vi "Write_NetworkStream_OCU_Override.vi"(0 "VKey":T1, 5 "Mainsail Position":T4, 7 "Jib Position":T3, 9 "Rudder Setpoint":T2 min=-0.95 max=0.95 scale=1.0..-1.0, 11 "error in (no error)":errorcluster, 12 "OverrideMode":T5) -> (4 "Main Position":T4, 6 "Jib Position":T3, 8 "Rudder Position":T2 min=-0.95 max=0.95 scale=1.0..-1.0, 10 "data string":string, 15 "error out":errorcluster)   [LabVIEW 2013]
doc: "Takes in the key value pressed and changes the value of the main sail, jib, and rudder accordingly with the following mapping of the arrow keys (ish):\n\n\"Page Up\" -- rudder right | \"Up\" -- Main out | \"Page Down\" -- Jib out\n\"Left\" -- rudder left | \"Down\" -- Main in | \"Right\" -- Jib in\n\nIt then bundles the main sail, jib sail, and rudder override commands and sends them to the boat using NetworkStreams. It also bundles with them the override mode so the Forebrain Sense can determine which actuator setting so implement and which to ignore. Deals with coersions, becaues humans can be silly.\n\n\n\nWritten by Victoria Coleman 04/12/14"
uses:
  cRIO_Code/Data/TypeDefs/Sail Set Suggestions.ctl
  cRIO_Code/Data/TypeDefs/OverrideMode.ctl
  cRIO_Code/Data/TypeDefs/MainsailPositionIndicator.ctl
  cRIO_Code/Data/TypeDefs/JibPositionIndicator.ctl
  cRIO_Code/Data/TypeDefs/Rudder Set Suggestions.ctl
  <vilib>/event_ctls.llb/eventvkey.ctl
  cRIO_Code/Data/TypeDefs/OverrideInformation.ctl
  OCU/CommandMessages.ctl
panel:
  in  "Sail Suggesstions":T6 {"MainSailSuggestion" min=0.0 max=1.0; "JibSailSuggestion" min=0.0 max=1.0}
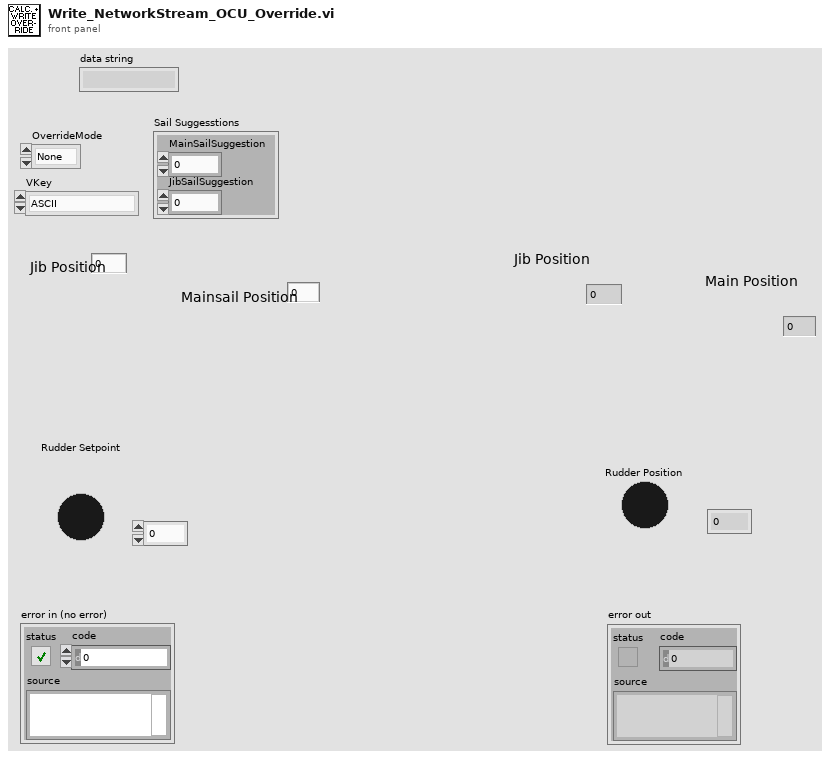
[diagram p1: front panel]
types:
  T1 = typedef "eventvkey.ctl" = enum16{"ASCII", "Enter", "Return", "Shift", "Ctrl", "Alt", "Cmd", "Opt", "Caps", "NumLock", "Clear", "Break", "Up", "Down", "Left", "Right", "Insert", "Delete", "Home", "End", "PageUp", "PageDown", "Escape", "Help", "Pause", "ScrollLock", "F1", "F2", "F3", "F4", "F5", "F6", "F7", "F8", "F9", "F10", "F11", "F12", "F13", "F14", "F15", "F16", "F17", "F18", "F19", "F20", "F21", "F22", "F23", "F24", "Play", "VolumeUp", "VolumeDown", "Mute", "Two Byte Char"}
  T2 = typedef "Rudder Set Suggestions.ctl" = dbl
  T3 = typedef "JibPositionIndicator.ctl" = dbl
  T4 = typedef "MainsailPositionIndicator.ctl" = dbl
  T5 = typedef "OverrideMode.ctl" = enum16{"None", "Rudder", "Sails", "Both"}
  T6 = typedef "Sail Set Suggestions.ctl" = cluster{"MainSailSuggestion":dbl, "JibSailSuggestion":dbl}
  T7 = typedef "OverrideInformation.ctl" = cluster{"OverrideMode":T5, "SailSetting":T6, "Rudder Setpoint":T2, "Sim_Wind_Speed":dbl, "Sim_Wind_Heading":dbl}
  T8 = typedef "CommandMessages.ctl" = enum16{"Pass", "OverrideMode", "Add mission", "Delete mission", "Change constants"}
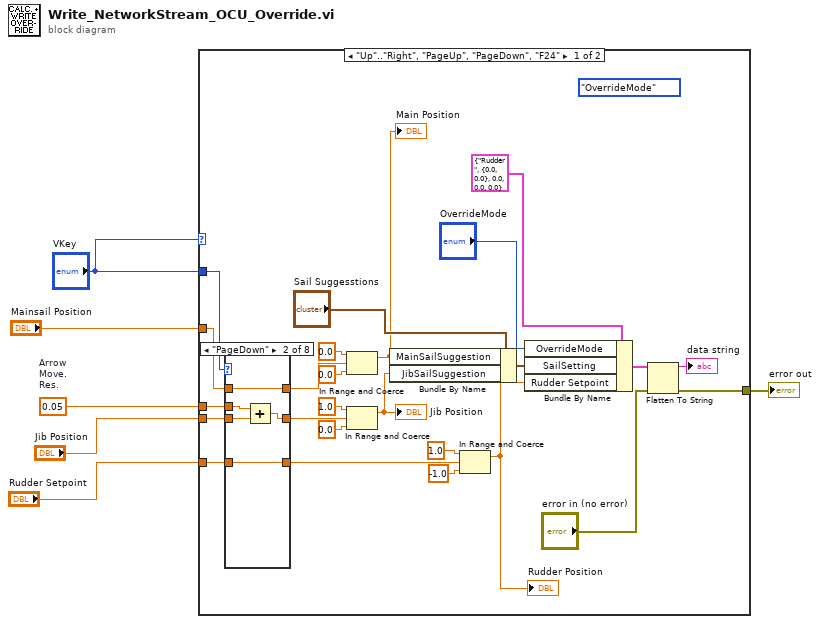
[diagram p0: block diagram]
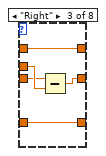
[diagram p3: hidden frame]
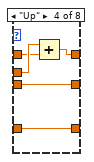
[diagram p4: hidden frame]
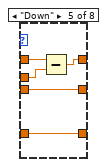
[diagram p5: hidden frame]
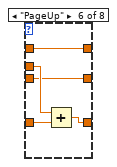
[diagram p6: hidden frame]
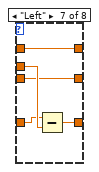
[diagram p7: hidden frame]
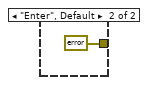
[diagram p9: hidden frame]
diagram:
  w6 = T4 0.05  # Arrow Move. Res.
  n1 = case shown="\"Up\"..\"Right\", \"PageUp\", \"PageDown\", \"F24\"" "VKey" {
    tunnel: w6 -> [w26 _]
    tunnel: "Jib Position" -> [w13 _]
    tunnel: "Rudder Setpoint" -> [w12 _]
    tunnel: [w8 errorcluster {"status"=FALSE, "code"=0, "source"=""} ("error out")] -> w3
    tunnel: "Mainsail Position" -> [w10 _]
    tunnel: "VKey" -> [w9 _]
    frame "Up".."Right", "PageUp", "PageDown", "F24" {
      (unwired) CommandMessages."OverrideMode" ("Commands")
      n2 = case shown="\"PageDown\"" w9 {
        tunnel: w12 -> [w32 w36 w42 w47 w51 w58 w63 w65]
        tunnel: w13 -> [w33 w38 w41 w45 w52 w57 w62 w66]
        tunnel: w10 -> [w34 w37 w40 w48 w54 w56 w61 w67]
        tunnel: w26 -> [_ w39 w44 w49 w53 w59 w64 _]
        tunnel: [w33 w35 w43 w45 w52 w57 w62 w66] -> w30
        tunnel: [w34 w37 w40 w46 w50 w56 w61 w67] -> w24
        tunnel: [w32 w36 w42 w47 w51 w55 w60 w65] -> w17
        frame "ASCII", Default {
        }
        frame "PageDown" {
          n3 = Add(x=w39, y=w38) -> (x+y=w35:T4)
        }
        frame "Right" {
          n4 = Subtract(x=w41, y=w44) -> (x-y=w43:T3)
        }
        frame "Up" {
          n5 = Add(x=w49, y=w48) -> (x+y=w46:T4)
        }
        frame "Down" {
          n6 = Subtract(x=w54, y=w53) -> (x-y=w50:T4)
        }
        frame "PageUp" {
          n7 = Add(x=w59, y=w58) -> (x+y=w55:T4)
        }
        frame "Left" {
          n8 = Subtract(x=w63, y=w64) -> (x-y=w60:T2)
        }
        frame "F24" {
        }
      }
      n9 = In Range and Coerce(upper limit=T4 0.0, x=w24, lower limit=T4 0.0) -> (coerced(x)=w19:T4)  [unwired: 1 out]
      "Main Position" <- w19
      n10 = In Range and Coerce(upper limit=T3 1.0, x=w30, lower limit=T3 0.0) -> (coerced(x)=w20:T3)  [unwired: 1 out]
      "Jib Position" <- w20
      n11 = Bundle By Name(cluster="Sail Suggesstions", "MainSailSuggestion"=w19, "JibSailSuggestion"=w20) -> (w22:T6)
      n12 = In Range and Coerce(upper limit=T2 1.0, x=w17, lower limit=T2 -1.0) -> (coerced(x)=w16:T2)  [unwired: 1 out]
      "Rudder Position" <- w16
      n13 = Bundle By Name(cluster=T7 {"OverrideMode"=enum."Rudder", "SailSetting"={"MainSailSuggestion"=0.0, "JibSailSuggestion"=0.0}, "Rudder Setpoint"=0.0, "Sim_Wind_Speed"=0.0, "Sim_Wind_Heading"=0.0} ("OverrideInfo"), "OverrideMode"="OverrideMode", "SailSetting"=w22, "Rudder Setpoint"=w16) -> (w21:T7)
      n14 = Flatten To String(anything=w21, error in (no error)="error in (no error)") -> (data string=→"data string":string, error out=w8:errorcluster)  [unwired: 2 in, 1 out]
    }
    frame "Enter", Default {
    }
  }
  "error out" <- w3
